vi "Create Query (array).vi"(5 "URI-Component.Query":refnum<class "URI-Component.Query.lvclass">, 8 "error in (no error)":errorcluster, 11 "Query":cluster{"argument":string, "value":string}[](array[cluster])) -> (0 "error out":errorcluster, 3 "URI-Component.Query":refnum<class "URI-Component.Query.lvclass">)   [LabVIEW 2013, in "openURI.lvlib" / "URI-Component.Query.lvclass"]
uses:
  URI-Component.Query.lvclass
  URI-Component.Query.lvclass/URI-Component.Query.ctl
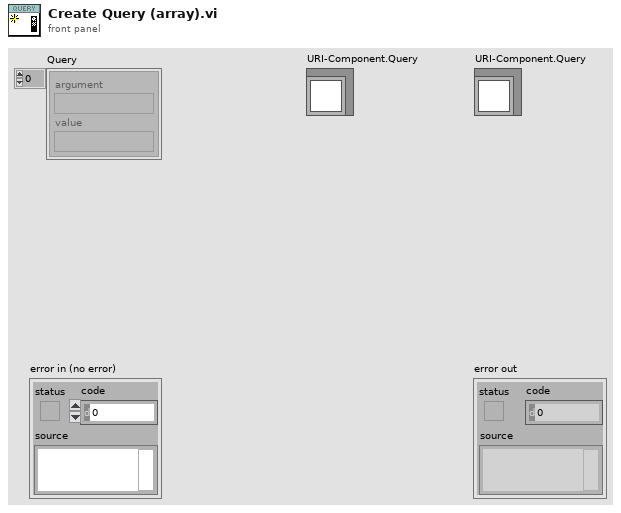
[diagram p1: front panel]
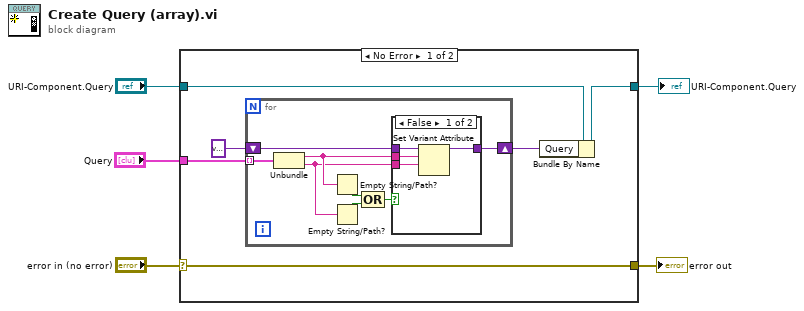
[diagram p0: block diagram]
diagram:
  n1 = case shown="No Error" "error in (no error)" {
    selector: "error in (no error)" -> [w6 w26]
    tunnel: [w6 w26] -> w4
    tunnel: [w7 w25] -> w2
    tunnel: "URI-Component.Query" -> [w8 w25]
    tunnel: "Query" -> [w9 _]
    frame No Error {
      n2 = for {
        shift-right: [w18] -> w10
        shift-left: variant ("variant") -> [w19]
        tunnel: w9 -> [w17] mode=indexing
        n3 = Unbundle(w17) -> ("argument"=w16:string, "value"=w15:string)
        n4 = Empty String/Path?(string/path=w16) -> (empty?=w13:bool)
        n5 = Empty String/Path?(string/path=w15) -> (empty?=w14:bool)
        n6 = Compound Arithmetic op=OR(w13, w14) -> (w12:bool)
        n7 = case shown="False" w12 {
          tunnel: w19 -> [w23 w24]
          tunnel: [w22 w24] -> w18
          tunnel: w16 -> [w21 _]
          tunnel: w15 -> [w20 _]
          frame False {
            n8 = Set Variant Attribute(Variant=w23, name=w21, value=w20) -> (Variant out=w22:variant)  [unwired: 1 in, 2 out]
          }
          frame True {
          }
        }
      }
      n9 = Bundle By Name(cluster=w8, "Query"=w10) -> (w7:refnum<class "URI-Component.Query.lvclass">)
    }
    frame Error {
    }
  }
  "error out" <- w4
  "URI-Component.Query" <- w2
